vi "Auto Number Create Table.vi"(8 "error in (no error)":errorcluster, 11 "Connection Refnum":T1) -> (0 "error out":errorcluster, 3 "Connection Refnum":T1)   [LabVIEW 2011]
uses:
  SI.LIB/ODBC/SQL Controls/Connection Refnum.ctl
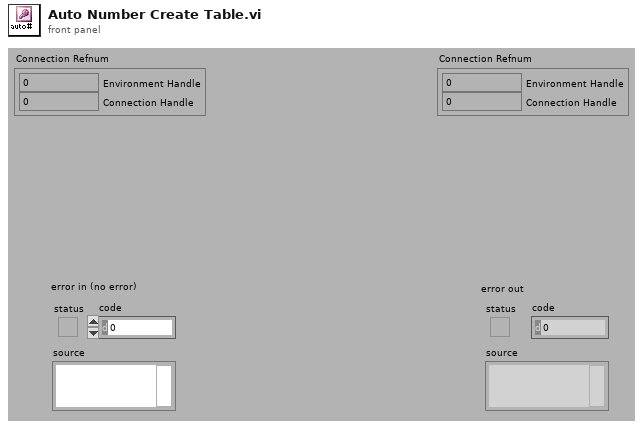
[diagram p1: front panel]
types:
  T1 = typedef "Connection Refnum.ctl" = cluster{"Environment Handle":i32, "Connection Handle":i32}
  T2 = typedef "Statement Refnum.ctl" = cluster{"Statement Handle":i32, "Parameter Number":u16}
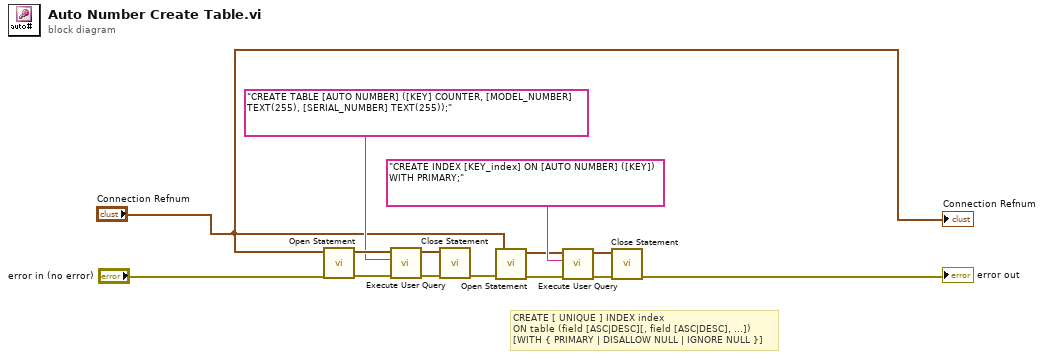
[diagram p0: block diagram]
diagram:
  # "CREATE [ UNIQUE ] INDEX index\nON table (field [ASC|DESC][, field [ASC|DESC], ...])\n[WITH { PRIMARY | DISALLOW NULL | IGNORE NULL }]"
  n1 = call "Open Statement.vi"("error in (no error)"="error in (no error)", "Connection Refnum"="Connection Refnum") -> ("error out"=w13:errorcluster, "Statement Refnum"=w14:T2)  [unwired: 4 out]
  n2 = call "Execute User Query.vi"("error in (no error)"=w13, "User Query"="CREATE TABLE [AUTO NUMBER] ([KEY] COUNTER, [MODEL_NUMBER] TEXT(255), [SERIAL_NUMBER] TEXT(255));" ("format string"), "Statement Refnum"=w14) -> ("error out"=w12:errorcluster, "Statement Refnum"=w11:T2)  [unwired: 1 in, 2 out]
  n3 = call "Close Statement.vi"("error in (no error)"=w12, "Statement Refnum"=w11) -> ("error out"=w7:errorcluster)  [unwired: 5 out]
  n4 = call "Open Statement.vi"("error in (no error)"=w7, "Connection Refnum"="Connection Refnum") -> ("error out"=w8:errorcluster, "Statement Refnum"=w5:T2)  [unwired: 4 out]
  n5 = call "Execute User Query.vi"("error in (no error)"=w8, "User Query"="CREATE INDEX [KEY_index] ON [AUTO NUMBER] ([KEY]) WITH PRIMARY;" ("format string"), "Statement Refnum"=w5) -> ("error out"=w9:errorcluster, "Statement Refnum"=w4:T2)  [unwired: 1 in, 2 out]
  n6 = call "Close Statement.vi"("error in (no error)"=w9, "Statement Refnum"=w4) -> ("error out"=→"error out":errorcluster)  [unwired: 5 out]
  "Connection Refnum" <- "Connection Refnum"
